vi "channel type to group string.vi"(11 "channel type":T1) -> (3 "FPGA.Controls":string)   [LabVIEW 2016]
uses:
  FPGA-Addon/Source/System Explorer/SubVIs/Channel Type.ctl
  FPGA-Addon/Source/System Explorer/FPGA Addon System Explorer.lvlib
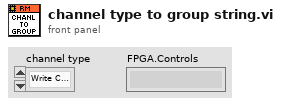
[diagram p1: front panel]
types:
  T1 = typedef "FPGA Addon System Explorer.lvlib/Channel Type.ctl" = enum16{"Write Channel", "Read Channel", "Write Waveform", "Read Waveform"}
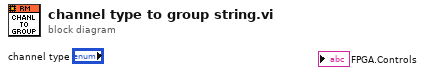
[diagram p0: block diagram]
diagram:
